vi "WS1050 VSA_Delta C Calculation.vi"(8 "error in (no error)":errorcluster, 10 "VSA_T":string[](array[string]), 11 "VSA_T0":string[](array[string])) -> (0 "error out":errorcluster, 2 "VSA Delta C(pF)":dbl[](array[numeric]), 3 "VSA Delta C(pF)":string[](array[string]))   [LabVIEW 2012]
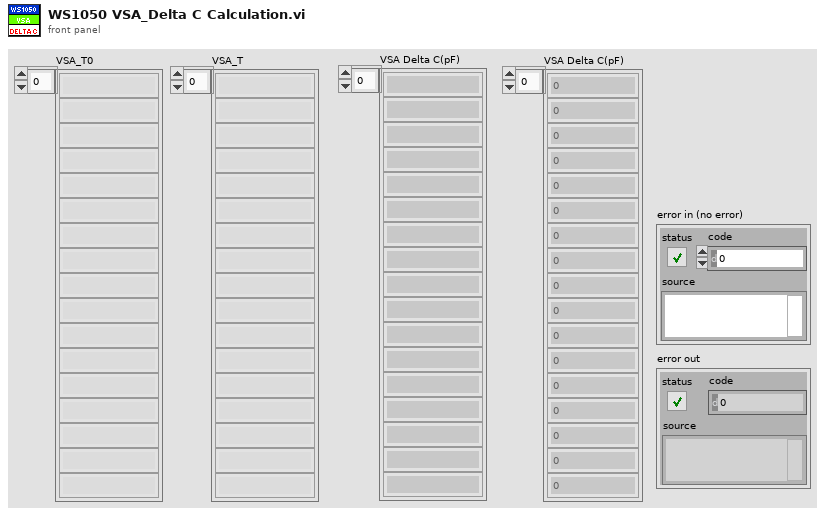
[diagram p1: front panel]
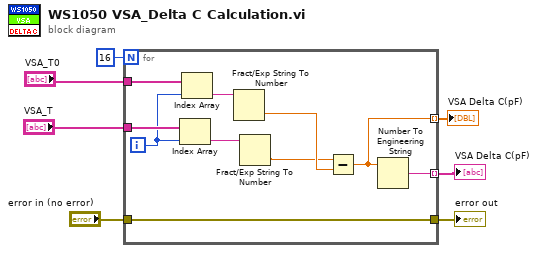
[diagram p0: block diagram]
diagram:
  n1 = for {
    N: 16 -> [_]
    tunnel: "VSA_T0" -> [w16]
    tunnel: "error in (no error)" -> [w15]
    tunnel: [w15] -> w6
    tunnel: "VSA_T" -> [w13]
    tunnel: [w10] -> w5 mode=indexing
    tunnel: [w8] -> w1 mode=indexing
    i -> [w9]
    n2 = Index Array(array=w13, index=w9) -> (element=w12:string)
    n3 = Index Array(array=w16, index=w9) -> (element=w17:string)
    n4 = Fract/Exp String To Number(string=w17) -> (number=w14:dbl)  [unwired: 3 in, 1 out]
    n5 = Fract/Exp String To Number(string=w12) -> (number=w11:dbl)  [unwired: 3 in, 1 out]
    n6 = Subtract(x=w11, y=w14) -> (x-y=w8:dbl)
    n7 = Number To Engineering String(4:w8) -> (0:w10:string)  [unwired: 3 in]
  }
  "error out" <- w6
  "VSA Delta C(pF)" <- w5
  "VSA Delta C(pF)" <- w1
